vi "Autonomous Independent.vi"() -> ()   [LabVIEW 2013]
doc: "This VI is called when autonomous begins, and will automatically be terminated when autonomous ends. You can carry out timed or sensor driven robot movement independently without needing to return to the caller."
uses:
  <vilib>/Rock Robotics/WPI/DriverStation/WPI_DriverStationMatch Info.ctl
  <vilib>/Rock Robotics/WPI/Solenoid/WPI_SolenoidValue.ctl
  <vilib>/Rock Robotics/WPI/Relay/WPI_RelayValue.ctl
  Robot Global Data.vi
  <vilib>/addons/control/pid/pid.llb/PID (DBL).vi
  <vilib>/Rock Robotics/WPI/Solenoid/WPI_SolenoidSetEnum.vi
  <vilib>/Rock Robotics/WPI/Joystick/WPI_JoystickGetSetRefNum.vi
  <vilib>/addons/control/pid/NI_PID_pid.lvlib
panel:
  in  "Angle to Move Left":dbl=-1.1
  in  "Angle to Move Right":dbl=1.1 format="%.2f"
  in  "Feet To Move Left":dbl=2.0
  in  "Feet To Move Right":dbl=2.0 format="%.2f"
  out "Reseting constant":bool
  in  "Threshold for shooter":dbl=0.015
  out "Ready To Fire":bool
  in  "PID gains":T1={"proportional gain (Kc)"=1.0, "integral time (Ti, min)"=0.007, "derivative time (Td, min)"=0.0} {"derivative time (Td, min)" format="%.3f"; "integral time (Ti, min)" format="%.3f"; "proportional gain (Kc)" format="%.3f"}
  in  "Maximum Encoder speed":dbl=25000.0
  out "Time Last Fired":dbl
  in  "Posistioned":string="Nothing"
  in  "S Wait Time":dbl=1200.0
  in  "S Fire Time":dbl=1400.0
  in  "Shooter Speed":dbl format="%.2f"
  in  "Shooter On":bool=TRUE
  in  "Match Info":T2={"Autonomous Elapsed Seconds"=0.0, "TeleOp Elapsed Seconds"=0.0, "Disabled Elapsed Seconds"=0.0, "Visited Autonomous"=FALSE, "Visited TeleOp"=FALSE, "Visited Disabled"=FALSE, "Autonomous Settings"={"Autonomous Style"=enum."Independent", "VI Refnum"=refnum}}
  out "Angle Target":dbl
  out "Distance From Target":dbl
  in  "Current Status":string="Roaming"
  # "Be sure to right-click and choose Data Operations>>Make Current Value default if you want to save the array values with the VI"
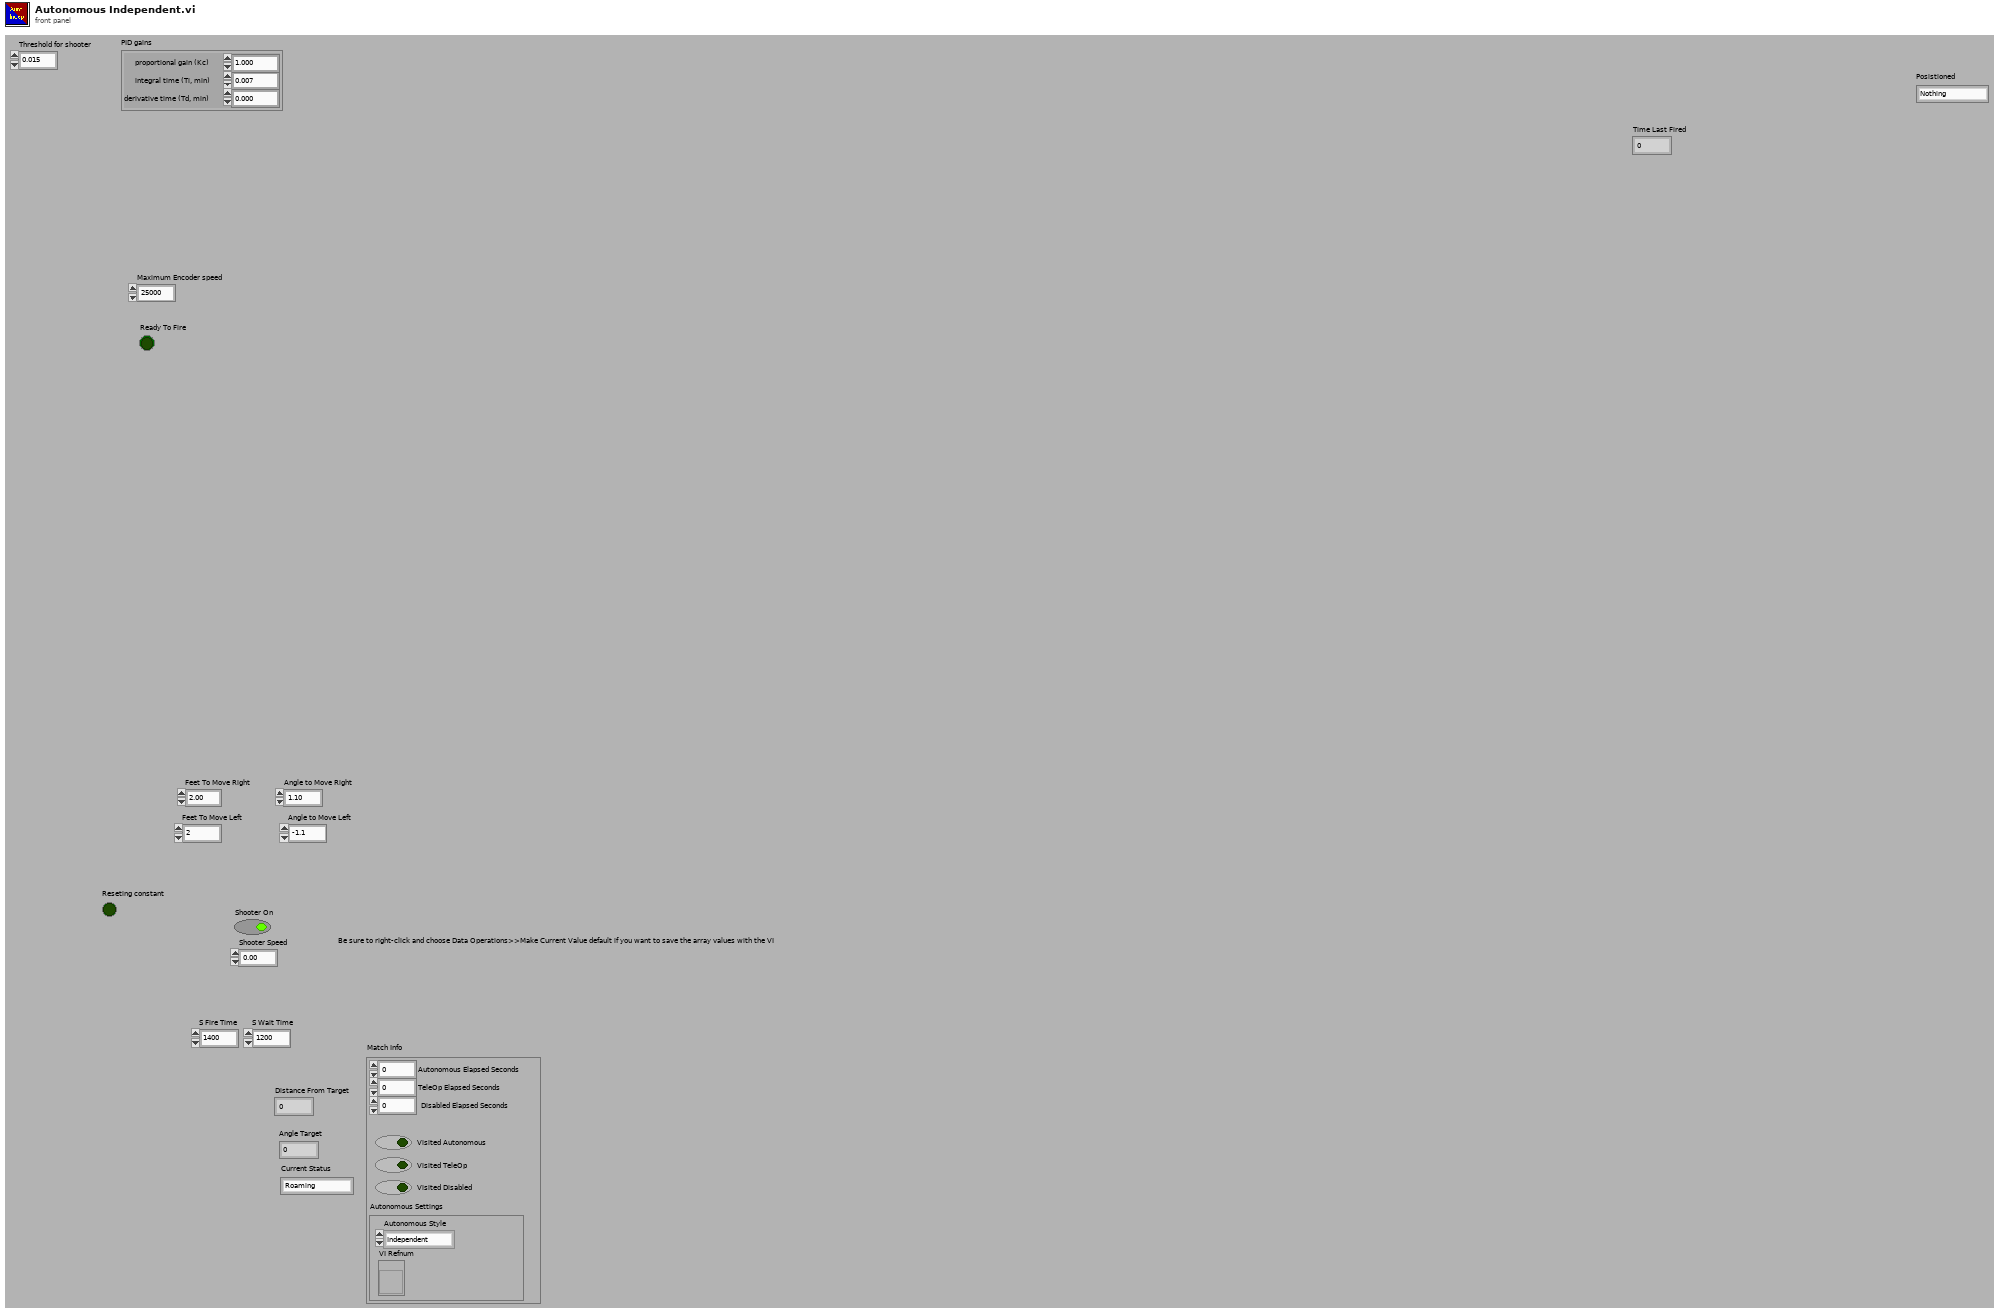
[diagram p1: front panel]
types:
  T1 = cluster{"proportional gain (Kc)":dbl, "integral time (Ti, min)":dbl, "derivative time (Td, min)":dbl}
  T2 = typedef "WPI_DriverStationMatch Info.ctl" = cluster{"Autonomous Elapsed Seconds":dbl, "TeleOp Elapsed Seconds":dbl, "Disabled Elapsed Seconds":dbl, "Visited Autonomous":bool, "Visited TeleOp":bool, "Visited Disabled":bool, "Autonomous Settings":cluster{"Autonomous Style":enum16{"Iterative", "Independent"}, "VI Refnum":refnum<vi>}}
  T3 = typedef "WPI_SolenoidValue.ctl" = enum16{"Off", "On", "Forward", "Reverse"}
  T4 = typedef "WPI_RelayValue.ctl" = enum16{"Off", "On", "Forward", "Reverse"}
  T5 = typedef "WPI_EncoderDevRef.ctl" = cluster{"DevStatus":errorcluster, "EncoderIndex":T6, "CounterIndex":T7, "DistancePerCount":dbl, "Decoding Type":T8}
  T6 = typedef "FPGA_EncoderIdx.ctl" = enum8{"Enc 0", "Enc 1", "Enc 2", "Enc 3", "Invalid"}
  T7 = typedef "FPGA_CounterCtrSystemIndex.ctl" = enum8{"Ctr 0", "Ctr 1", "Ctr 2", "Ctr 3", "Ctr 4", "Ctr 5", "Ctr 6", "Ctr 7", "Invalid"}
  T8 = typedef "WPI_EncoderType.ctl" = enum16{"1x", "2x", "4x"}
  T9 = typedef "WPI_RelayDevRef.ctl" = cluster{"DevStatus":errorcluster, "Relay Channel":T10, "Digital Module":T11, "Relay Direction":T12}
  T10 = typedef "FPGA_DIORelayChannel.ctl" = enum8{"Relay 1", "Relay 2", "Relay 3", "Relay 4", "Relay 5", "Relay 6", "Relay 7", "Relay 8", "Invalid"}
  T11 = typedef "FPGA_TypedefDigitalModule.ctl" = enum16{"Digital Module 1", "Digital Module 2"}
  T12 = typedef "WPI_RelayDirection.ctl" = enum16{"Both directions", "Forward only", "Reverse only"}
  T13 = typedef "WPI_SolenoidDevRef.ctl" = cluster{"DevStatus":errorcluster, "Solenoid Module":T14, "Forward Solenoid Channel":T15, "Reverse Solenoid Channel":T15}
  T14 = typedef "FPGA_TypedefSolenoidModule.ctl" = enum16{"Solenoid Module 1", "Solenoid Module 2"}
  T15 = typedef "WPI_SolenoidChannel.ctl" = enum8{"Solenoid 1", "Solenoid 2", "Solenoid 3", "Solenoid 4", "Solenoid 5", "Solenoid 6", "Solenoid 7", "Solenoid 8", "Invalid"}
  T16 = cluster{"Center Position":cluster{"X":dbl, "Y":dbl}, "Distance (ft)":dbl, "Center":bool}[]
  T17 = cluster{"Center Position":cluster{"X":dbl, "Y":dbl}, "Distance (ft)":dbl, "Center":bool}
  T18 = typedef "WPI_MotorControlDeviceRef.ctl" = cluster{"DeviceStatus":errorcluster, "Type":enum16{"PWM", "CAN"}, "PWM":cluster{"Digital Module":T11, "PWM Channel":T19, "DeadBand":T20}, "CAN":cluster{"Device Number":u8, "Control Mode":T21, "Semaphore":T22, "Max Vout":dbl}, "Invert":bool, "TransformRef":T23, "InvTransformRef":T23}
  T19 = typedef "FPGA_DIOPWMChannel.ctl" = enum8{"PWM 1", "PWM 2", "PWM 3", "PWM 4", "PWM 5", "PWM 6", "PWM 7", "PWM 8", "PWM 9", "PWM 10", "Invalid"}
  T20 = typedef "WPI_PWMDeadband.ctl" = cluster{"Name":string, "maxPositivePwm":i32, "minPositivePwm":i32, "centerPwm":i32, "maxNegativePwm":i32, "minNegativePwm":i32, "angularRange":u16}
  T21 = typedef "WPI_CANJaguar_ControlMode.ctl" = enum8{"Percent VBus", "Current", "Speed", "Position", "Voltage"}
  T22 = typedef "Semaphore RefNum" = refnum<k1>
  T23 = typedef "WPI_PWMTransform_ConPane.ctl" = refnum<vi>
  T24 = typedef "WPI_JoystickDevRef.ctl" = cluster{"Device":T25}
  T25 = typedef "WPI_JoystickDeviceEnum.ctl" = enum16{"USB 1", "USB 2", "USB 3", "USB 4", "Kinect 1", "Kinect 2"}
  T26 = cluster{"axis 1 (x)":dbl, "axis 2 (y)":dbl, "axis 3 (throttle)":dbl, "axis 4":dbl, "axis 5":dbl, "axis 6":dbl}
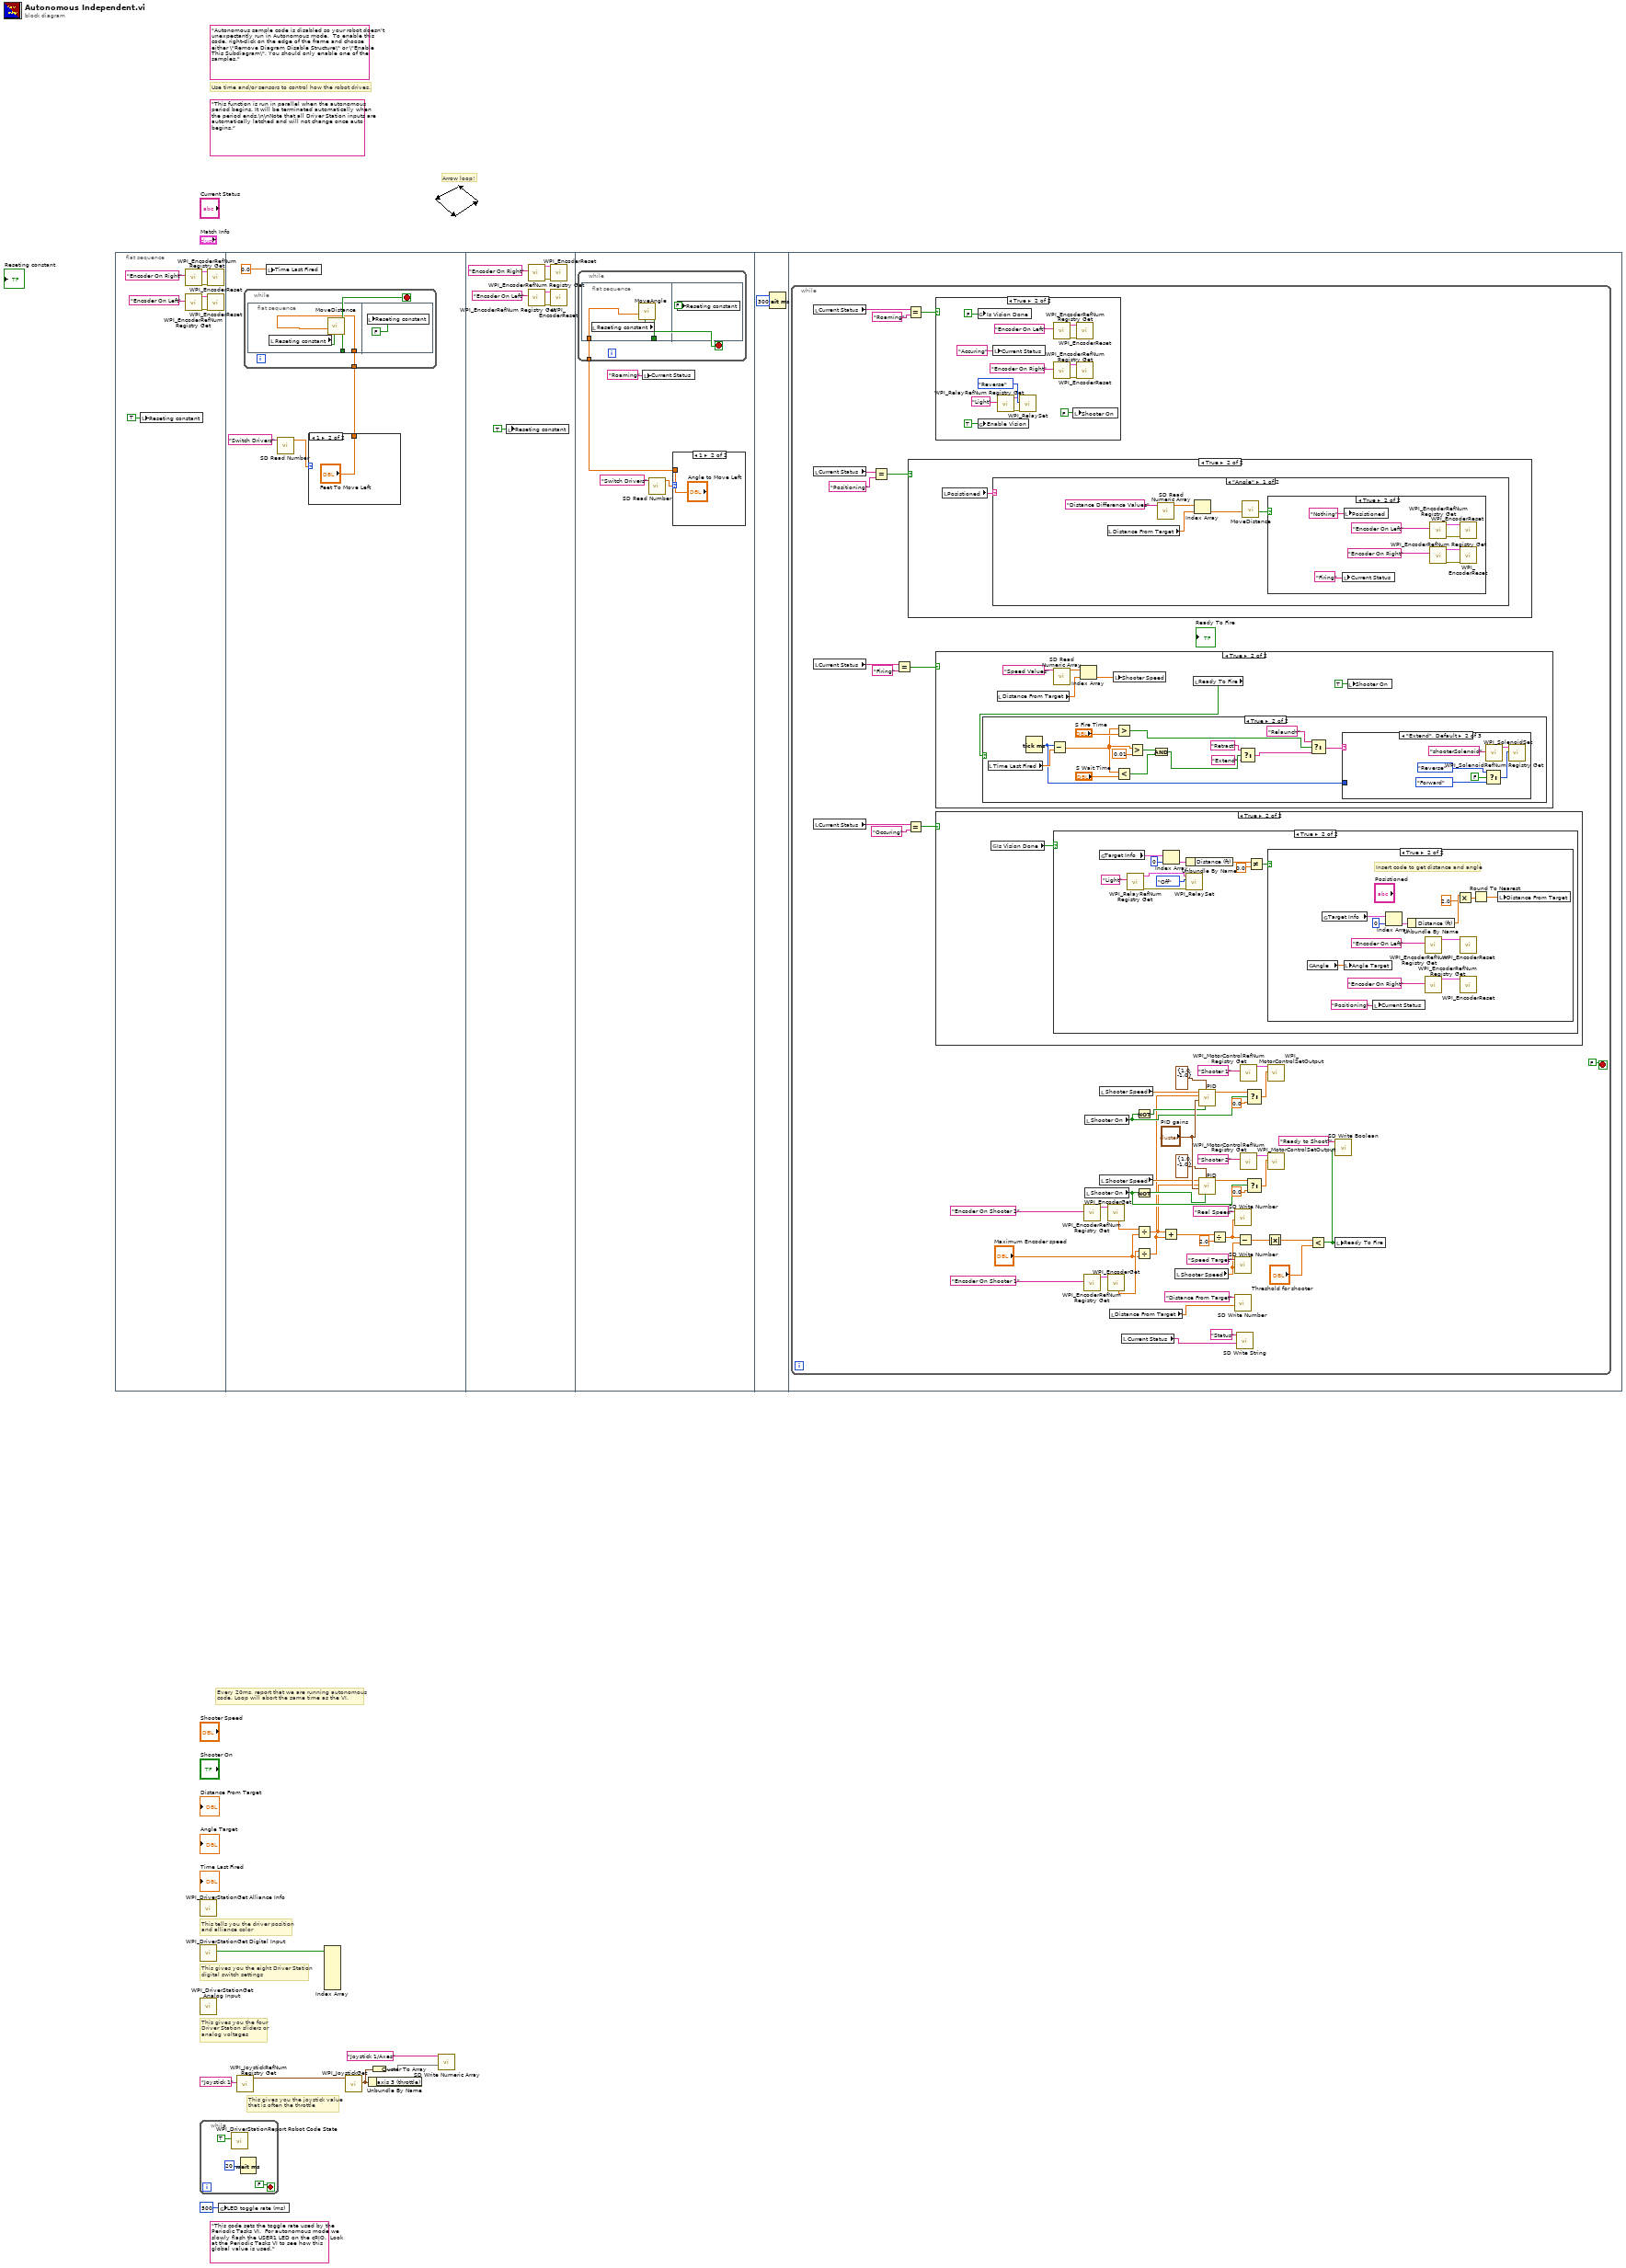
[diagram p0: block diagram]
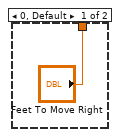
[diagram p2: hidden frame]
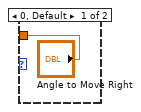
[diagram p3: hidden frame]
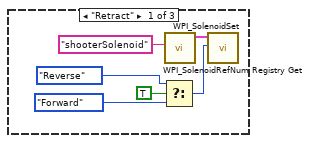
[diagram p6: hidden frame]
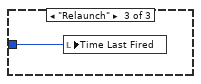
[diagram p7: hidden frame]
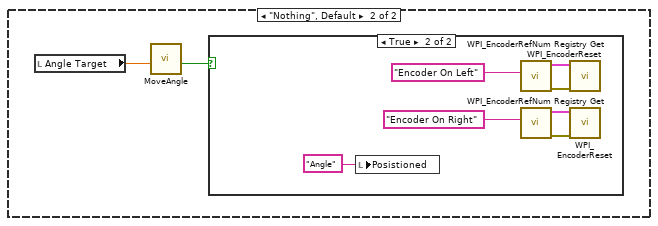
[diagram p11: hidden frame]
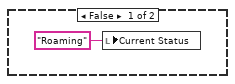
[diagram p15: hidden frame]
diagram:
  (unwired) "This code sets the toggle rate used by the Periodic Tasks VI.  For autonomous mode we slowly flash the USER1 LED on the cRIO.  Look at the Periodic Tasks VI to see how this global value is used."
  (unwired) "Autonomous sample code is disabled so your robot doesn't unexpectantly run in Autonomous mode.  To enable this code, right-click on the edge of the frame and choose either \"Remove Diagram Disable Structure\" or \"Enable This Subdiagram\". You should only enable one of the samples."
  (unwired) "This function is run in parallel when the autonomous period begins. It will be terminated automatically when the period ends.\n\nNote that all Driver Station inputs are automatically latched and will not change once auto begins."
  # "Arrow loop!"
  # "Every 20ms, report that we are running autonomous\ncode. Loop will abort the same time as the VI."
  # "This gives you the joystick value\nthat is often the throttle"
  # "Use time and/or sensors to control how the robot drives."
  # "This tells you the driver position\nand alliance color"
  # "This gives you the eight Driver Station\ndigital switch settings"
  # "This gives you the four\nDriver Station sliders or\nanalog voltages"
  n1 = flat-sequence {
    frame #0 {
      n2 = local write "Reseting constant"(TRUE ("Reseting constant")) -> ()
      n3 = call <vilib>:"WPI_EncoderRefNum Registry Get.vi"("refnum name"="Encoder On Right") -> ("error out"=w9:errorcluster, "EncoderDevRef"=w10:T5)  [unwired: 9 in]
      n4 = call <vilib>:"WPI_EncoderRefNum Registry Get.vi"("refnum name"="Encoder On Left") -> ("error out"=w11:errorcluster, "EncoderDevRef"=w12:T5)  [unwired: 9 in]
      n5 = call <vilib>:"WPI_EncoderReset.vi"("error in (no error)"=w9, "EncoderDevRef"=w10) -> ()  [unwired: 8 in, 2 out]
      n6 = call <vilib>:"WPI_EncoderReset.vi"("error in (no error)"=w11, "EncoderDevRef"=w12) -> ()  [unwired: 8 in, 2 out]
    }
    frame #1 {
      n7 = local write "Time Last Fired"(0.0 ("Time Last Fired")) -> ()
      n8 = call <vilib>:"SD Read Number.vi"("Name"="Switch Drivers") -> ("Numeric"=w16:dbl)  [unwired: 8 in, 2 out]
      n9 = case shown="1" w16 {
        tunnel: ["Feet To Move Right" "Feet To Move Left"] -> w15
        frame 0, Default {
        }
        frame 1 {
        }
      }
      n10 = while {
        tunnel: w15 -> [w21]
        stop <- w22 stop-if-true
        n11 = flat-sequence {
          tunnel: [w25] -> w22
          tunnel: w21 -> [w23]
          frame #0 {
            n12 = local read "Reseting constant"() -> (w24:bool)
            n13 = call "MoveDistance.vi"("reinitialize? (F)"=w24, "Distance From Target"=w23) -> ("Done?"=w25:bool)  [unwired: 9 in]
          }
          frame #1 {
            n14 = local write "Reseting constant"(FALSE ("Reseting constant")) -> ()
          }
        }
      }
    }
    frame #2 {
      n15 = local write "Reseting constant"(TRUE ("Reseting constant")) -> ()
      n16 = call <vilib>:"WPI_EncoderRefNum Registry Get.vi"("refnum name"="Encoder On Right") -> ("error out"=w33:errorcluster, "EncoderDevRef"=w32:T5)  [unwired: 9 in]
      n17 = call <vilib>:"WPI_EncoderRefNum Registry Get.vi"("refnum name"="Encoder On Left") -> ("error out"=w31:errorcluster, "EncoderDevRef"=w30:T5)  [unwired: 9 in]
      n18 = call <vilib>:"WPI_EncoderReset.vi"("error in (no error)"=w33, "EncoderDevRef"=w32) -> ()  [unwired: 8 in, 2 out]
      n19 = call <vilib>:"WPI_EncoderReset.vi"("error in (no error)"=w31, "EncoderDevRef"=w30) -> ()  [unwired: 8 in, 2 out]
    }
    frame #3 {
      n20 = local write "Current Status"("Roaming" ("Current Status")) -> ()
      n21 = call <vilib>:"SD Read Number.vi"("Name"="Switch Drivers") -> ("Numeric"=w35:dbl)  [unwired: 8 in, 2 out]
      n22 = case shown="1" w35 {
        tunnel: ["Angle to Move Right" "Angle to Move Left"] -> w34
        frame 0, Default {
        }
        frame 1 {
        }
      }
      n23 = while {
        tunnel: w34 -> [w40]
        stop <- w41 stop-if-true
        n24 = flat-sequence {
          tunnel: [w44] -> w41
          tunnel: w40 -> [w42]
          frame #0 {
            n25 = local read "Reseting constant"() -> (w43:bool)
            n26 = call "MoveAngle.vi"("reinitialize? (F)"=w43, "Angle Target"=w42) -> ("Done?"=w44:bool)  [unwired: 9 in]
          }
          frame #1 {
            n27 = local write "Reseting constant"(FALSE ("Reseting constant")) -> ()
          }
        }
      }
    }
    frame #4 {
      n28 = Wait (ms)(milliseconds to wait=u32 300) -> ()  [unwired: 1 out]
    }
    frame #5 {
      n29 = while {
        stop <- FALSE stop-if-true
        n30 = local read "Current Status"() -> (w94:string)
        n31 = local read "Current Status"() -> (w98:string)
        n32 = local read "Current Status"() -> (w91:string)
        n33 = local read "Current Status"() -> (w102:string)
        n34 = Equal?(x=w98, y="Positioning") -> (x = y?=w96:bool)
        n35 = Equal?(x=w91, y="Firing") -> (x = y?=w92:bool)
        n36 = Equal?(x=w94, y="Roaming") -> (x = y?=w93:bool)
        n37 = Equal?(x=w102, y="Occuring") -> (x = y?=w100:bool)
        n38 = case shown="True" w96 {
          frame False {
          }
          frame True {
            n39 = local read "Posistioned"() -> (w151:string)
            n40 = case shown="\"Angle\"" w151 {
              frame "Angle" {
                n41 = local read "Distance From Target"() -> (w154:dbl)
                n42 = call <vilib>:"SD Read Numeric Array.vi"("Name"="Distance Difference Values") -> ("Numeric Array"=w156:dbl[])  [unwired: 8 in, 2 out]
                n43 = Index Array(array=w156, index=w154) -> (element=w153:dbl)
                n44 = call "MoveDistance.vi"("Distance From Target"=w153) -> ("Done?"=w152:bool)  [unwired: 10 in]
                n45 = case shown="True" w152 {
                  frame False {
                  }
                  frame True {
                    n46 = local write "Current Status"("Firing" ("Current Status")) -> ()
                    n47 = local write "Posistioned"("Nothing" ("Posistioned")) -> ()
                    n48 = call <vilib>:"WPI_EncoderRefNum Registry Get.vi"("refnum name"="Encoder On Left") -> ("error out"=w160:errorcluster, "EncoderDevRef"=w161:T5)  [unwired: 9 in]
                    n49 = call <vilib>:"WPI_EncoderRefNum Registry Get.vi"("refnum name"="Encoder On Right") -> ("error out"=w162:errorcluster, "EncoderDevRef"=w163:T5)  [unwired: 9 in]
                    n50 = call <vilib>:"WPI_EncoderReset.vi"("error in (no error)"=w160, "EncoderDevRef"=w161) -> ()  [unwired: 8 in, 2 out]
                    n51 = call <vilib>:"WPI_EncoderReset.vi"("error in (no error)"=w162, "EncoderDevRef"=w163) -> ()  [unwired: 8 in, 2 out]
                  }
                }
              }
              frame "Nothing", Default {
                n52 = local read "Angle Target"() -> (w166:dbl)
                n53 = call "MoveAngle.vi"("Angle Target"=w166) -> ("Done?"=w165:bool)  [unwired: 10 in]
                n54 = case shown="True" w165 {
                  frame False {
                  }
                  frame True {
                    n55 = local write "Posistioned"("Angle" ("Posistioned")) -> ()
                    n56 = call <vilib>:"WPI_EncoderRefNum Registry Get.vi"("refnum name"="Encoder On Left") -> ("error out"=w171:errorcluster, "EncoderDevRef"=w170:T5)  [unwired: 9 in]
                    n57 = call <vilib>:"WPI_EncoderRefNum Registry Get.vi"("refnum name"="Encoder On Right") -> ("error out"=w169:errorcluster, "EncoderDevRef"=w168:T5)  [unwired: 9 in]
                    n58 = call <vilib>:"WPI_EncoderReset.vi"("error in (no error)"=w171, "EncoderDevRef"=w170) -> ()  [unwired: 8 in, 2 out]
                    n59 = call <vilib>:"WPI_EncoderReset.vi"("error in (no error)"=w169, "EncoderDevRef"=w168) -> ()  [unwired: 8 in, 2 out]
                  }
                }
              }
            }
          }
        }
        n60 = case shown="True" w93 {
          frame False {
          }
          frame True {
            n61 = global write "Robot Global Data.vi" "Is Vision Done"(FALSE ("Is Vision Done")) -> ()
            n62 = global write "Robot Global Data.vi" "Enable Vision"(TRUE ("Enable Vision")) -> ()
            n63 = local write "Current Status"("Accuring" ("Current Status")) -> ()
            n64 = call <vilib>:"WPI_RelayRefNum Registry Get.vi"("refnum name"="Light") -> ("error out"=w148:errorcluster, "RelayDevRef"=w147:T9)  [unwired: 9 in]
            n65 = call <vilib>:"WPI_RelaySet.vi"("error in (no error)"=w148, "RelayValue"=WPI_RelayValue."Reverse", "RelayDevRef"=w147) -> ()  [unwired: 7 in, 2 out]
            n66 = call <vilib>:"WPI_EncoderRefNum Registry Get.vi"("refnum name"="Encoder On Left") -> ("error out"=w142:errorcluster, "EncoderDevRef"=w141:T5)  [unwired: 9 in]
            n67 = call <vilib>:"WPI_EncoderRefNum Registry Get.vi"("refnum name"="Encoder On Right") -> ("error out"=w144:errorcluster, "EncoderDevRef"=w143:T5)  [unwired: 9 in]
            n68 = local write "Shooter On"(FALSE ("Shooter On")) -> ()
            n69 = call <vilib>:"WPI_EncoderReset.vi"("error in (no error)"=w142, "EncoderDevRef"=w141) -> ()  [unwired: 8 in, 2 out]
            n70 = call <vilib>:"WPI_EncoderReset.vi"("error in (no error)"=w144, "EncoderDevRef"=w143) -> ()  [unwired: 8 in, 2 out]
          }
        }
        n71 = case shown="True" w92 {
          frame False {
          }
          frame True {
            n72 = local read "Distance From Target"() -> (w105:dbl)
            n73 = call <vilib>:"SD Read Numeric Array.vi"("Name"="Speed Values") -> ("Numeric Array"=w107:dbl[])  [unwired: 8 in, 2 out]
            n74 = Index Array(array=w107, index=w105) -> (element=w106:dbl)
            n75 = local write "Shooter Speed"(w106) -> ()
            n76 = local read "Ready To Fire"() -> (w104:bool)
            n77 = case shown="True" w104 {
              frame False {
              }
              frame True {
                n78 = local read "Time Last Fired"() -> (w123:dbl)
                n79 = Tick Count (ms)() -> (millisecond timer value=w111:u32)
                n80 = Subtract(x=w111, y=w123) -> (x-y=w116:dbl)
                n81 = Greater?(x=w116, y="S Fire Time") -> (0:w119:bool)
                n82 = Less?(x=w116, y="S Wait Time") -> (x < y?=w113:bool)
                n83 = Greater?(x=w116, y=0.01) -> (0:w114:bool)
                n84 = And(x=w114, y=w113) -> (x .and. y?=w112:bool)
                n85 = Select(t="Retract" ("f"), s=w112, f="Extend") -> (s? t:f=w117:string)
                n86 = Select(t="Relaunch" ("f"), s=w119, f=w117) -> (s? t:f=w121:string)
                n87 = case shown="\"Extend\", Default" w121 {
                  tunnel: w111 -> [_ _ w136]
                  frame "Retract" {
                    n88 = Select(t=WPI_SolenoidValue."Reverse" ("Value"), s=TRUE, f=WPI_SolenoidValue."Forward" ("Value")) -> (s? t:f=w128:T3)
                    n89 = call <vilib>:"WPI_SolenoidRefNum Registry Get.vi"("refnum name"="shooterSolenoid") -> ("SolenoidDevRef"=w124:T13)  [unwired: 9 in, 1 out]
                    n90 = call-poly <vilib>:"WPI_SolenoidSet.vi"("Value"=w128, "SolenoidDevRef"=w124) -> ()  [unwired: 8 in, 2 out]
                  }
                  frame "Extend", Default {
                    n91 = Select(t=WPI_SolenoidValue."Reverse" ("Value"), s=FALSE, f=WPI_SolenoidValue."Forward" ("Value")) -> (s? t:f=w134:T3)
                    n92 = call <vilib>:"WPI_SolenoidRefNum Registry Get.vi"("refnum name"="shooterSolenoid") -> ("SolenoidDevRef"=w130:T13)  [unwired: 9 in, 1 out]
                    n93 = call-poly <vilib>:"WPI_SolenoidSet.vi"("Value"=w134, "SolenoidDevRef"=w130) -> ()  [unwired: 8 in, 2 out]
                  }
                  frame "Relaunch" {
                    n94 = local write "Time Last Fired"(w136) -> ()
                  }
                }
              }
            }
            n95 = local write "Shooter On"(TRUE ("Shooter On")) -> ()
          }
        }
        n96 = case shown="True" w100 {
          frame False {
          }
          frame True {
            n97 = global read "Robot Global Data.vi" "Is Vision Done"() -> (w174:bool)
            n98 = case shown="True" w174 {
              frame False {
              }
              frame True {
                n99 = global read "Robot Global Data.vi" "Target Info"() -> (w184:T16)
                n100 = call <vilib>:"WPI_RelayRefNum Registry Get.vi"("refnum name"="Light") -> ("error out"=w177:errorcluster, "RelayDevRef"=w178:T9)  [unwired: 9 in]
                n101 = Index Array(array=w184, index=0) -> (element=w182:T17)
                n102 = Unbundle By Name(w182) -> ("Distance (ft)"=w180:dbl)
                n103 = call <vilib>:"WPI_RelaySet.vi"("error in (no error)"=w177, "RelayValue"=WPI_RelayValue."Off", "RelayDevRef"=w178) -> ()  [unwired: 7 in, 2 out]
                n104 = Not Equal?(x=w180, y=0.0) -> (x != y?=w181:bool)
                n105 = case shown="True" w181 {
                  frame False {
                    n106 = local write "Current Status"("Roaming" ("Current Status")) -> ()
                  }
                  frame True {
                    # "Insert code to get distance and angle"
                    n107 = global read "Robot Global Data.vi" "Angle"() -> (w193:dbl)
                    n108 = global read "Robot Global Data.vi" "Target Info"() -> (w192:T16)
                    n109 = local write "Angle Target"(w193) -> ()
                    n110 = local write "Current Status"("Positioning" ("Current Status")) -> ()
                    n111 = Index Array(array=w192, index=0) -> (element=w190:T17)
                    n112 = Unbundle By Name(w190) -> ("Distance (ft)"=w188:dbl)
                    n113 = call <vilib>:"WPI_EncoderRefNum Registry Get.vi"("refnum name"="Encoder On Left") -> ("EncoderDevRef"=w196:T5)  [unwired: 9 in, 1 out]
                    n114 = call <vilib>:"WPI_EncoderRefNum Registry Get.vi"("refnum name"="Encoder On Right") -> ("EncoderDevRef"=w195:T5)  [unwired: 9 in, 1 out]
                    n115 = Multiply(x=w188, y=2.0) -> (x*y=w186:dbl)
                    n116 = call <vilib>:"WPI_EncoderReset.vi"("EncoderDevRef"=w196) -> ()  [unwired: 9 in, 2 out]
                    n117 = call <vilib>:"WPI_EncoderReset.vi"("EncoderDevRef"=w195) -> ()  [unwired: 9 in, 2 out]
                    n118 = Round To Nearest(number=w186) -> (nearest integer value=w189:dbl)
                    n119 = local write "Distance From Target"(w189) -> ()
                  }
                }
              }
            }
          }
        }
        n120 = call <vilib>:"WPI_EncoderRefNum Registry Get.vi"("refnum name"="Encoder On Shooter 2") -> ("EncoderDevRef"=w77:T5)  [unwired: 9 in, 1 out]
        n121 = call <vilib>:"WPI_EncoderRefNum Registry Get.vi"("refnum name"="Encoder On Shooter 1") -> ("EncoderDevRef"=w86:T5)  [unwired: 9 in, 1 out]
        n122 = local read "Shooter On"() -> (w66:bool)
        n123 = local read "Shooter On"() -> (w67:bool)
        n124 = local read "Shooter Speed"() -> (w65:dbl)
        n125 = local read "Shooter Speed"() -> (w64:dbl)
        n126 = call <vilib>:"WPI_EncoderGet.vi"("EncoderDevRef"=w77) -> ("Rate"=w69:dbl)  [unwired: 5 in, 5 out]
        n127 = call <vilib>:"WPI_EncoderGet.vi"("EncoderDevRef"=w86) -> ("Rate"=w70:dbl)  [unwired: 5 in, 5 out]
        n128 = local read "Distance From Target"() -> (w48:dbl)
        n129 = local read "Current Status"() -> (w47:string)
        n130 = Not(x=w66) -> (.not. x?=w88:bool)
        n131 = Not(x=w67) -> (.not. x?=w79:bool)
        n132 = Divide(x=w69, y="Maximum Encoder speed") -> (x/y=w62:dbl)
        n133 = Divide(x=w70, y="Maximum Encoder speed") -> (x/y=w61:dbl)
        n134 = Add(x=w62, y=w61) -> (x+y=w60:dbl)
        n135 = local read "Shooter Speed"() -> (w57:dbl)
        n136 = call-poly <vilib>:"PID.vi"("reinitialize? (F)"=w88, "output range"=cluster{"output high":dbl, "output low":dbl} {"output high"=1.0, "output low"=-1.0}, "PID gains"="PID gains", "process variable"=w61, "setpoint"=w65) -> ("output"=w87:dbl)  [unwired: 5 in, 1 out]
        n137 = call-poly <vilib>:"PID.vi"("reinitialize? (F)"=w79, "output range"=cluster{"output high":dbl, "output low":dbl} {"output high"=1.0, "output low"=-1.0}, "PID gains"="PID gains", "process variable"=w62, "setpoint"=w64) -> ("output"=w78:dbl)  [unwired: 5 in, 1 out]
        n138 = Divide(x=w60, y=2.0) -> (x/y=w56:dbl)
        n139 = call <vilib>:"SD Write Number.vi"("Numeric"=w48, "Name"="Distance From Target") -> ()  [unwired: 8 in, 2 out]
        n140 = call <vilib>:"SD Write Number.vi"("Numeric"=w56, "Name"="Real Speed") -> ()  [unwired: 8 in, 2 out]
        n141 = call <vilib>:"SD Write Number.vi"("Numeric"=w57, "Name"="Speed Target") -> ()  [unwired: 8 in, 2 out]
        n142 = call <vilib>:"SD Write String.vi"("String"=w47, "Name"="Status") -> ()  [unwired: 8 in, 2 out]
        n143 = Subtract(x=w56, y=w57) -> (x-y=w55:dbl)
        n144 = call <vilib>:"WPI_MotorControlRefNum Registry Get.vi"("refnum name"="Shooter 1") -> ("MotorControlDevRef"=w81:T18)  [unwired: 9 in, 1 out]
        n145 = call <vilib>:"WPI_MotorControlRefNum Registry Get.vi"("refnum name"="Shooter 2") -> ("MotorControlDevRef"=w72:T18)  [unwired: 9 in, 1 out]
        n146 = Select(t=w87, s=w66, f=0.0) -> (s? t:f=w83:dbl)
        n147 = Select(t=w78, s=w67, f=0.0) -> (s? t:f=w74:dbl)
        n148 = Absolute Value(x=w55) -> (abs(x)=w54:dbl)
        n149 = call <vilib>:"WPI_MotorControlSetOutput.vi"("Output"=w83, "MotorControlDevRef"=w81) -> ()  [unwired: 7 in, 3 out]
        n150 = call <vilib>:"WPI_MotorControlSetOutput.vi"("Output"=w74, "MotorControlDevRef"=w72) -> ()  [unwired: 7 in, 3 out]
        n151 = Less?(x=w54, y="Threshold for shooter") -> (x < y?=w52:bool)
        n152 = call <vilib>:"SD Write Boolean.vi"("Boolean"=w52, "Name"="Ready to Shoot?") -> ()  [unwired: 8 in, 2 out]
        n153 = local write "Ready To Fire"(w52) -> ()
      }
    }
  }
  n154 = call <vilib>:"WPI_DriverStationGet Alliance Info.vi"() -> ()  [unwired: 12 out]
  n155 = call <vilib>:"WPI_DriverStationGet Digital Input.vi"() -> ("Driver Station Digital Input (1-8)"=w7:bool[])  [unwired: 11 out]
  n156 = call <vilib>:"WPI_DriverStationGet Analog Input.vi"() -> ()  [unwired: 12 out]
  n157 = while {
    stop <- FALSE stop-if-true
    n158 = call <vilib>:"WPI_DriverStationReport Robot Code State.vi"("Autonomous"=TRUE) -> ()  [unwired: 10 in, 1 out]
    n159 = Wait (ms)(milliseconds to wait=u32 20) -> ()  [unwired: 1 out]
  }
  n160 = global write "Robot Global Data.vi" "LED toggle rate (ms)"(u32 500 ("LED ms toggle rate")) -> ()
  n161 = call <vilib>:"WPI_JoystickRefNum Registry Get.vi"("refnum name"="Joystick 1") -> ("JoystickDevRef"=w5:T24)  [unwired: 1 in, 9 out]
  n162 = Index Array(array=w7) -> ()  [unwired: 8 in, 8 out]
  n163 = call <vilib>:"WPI_JoystickGet.vi"("JoystickDevRef"=w5) -> ("Axes"=w2:T26)  [unwired: 1 in, 5 out]
  n164 = Unbundle By Name(w2) -> ()  [unwired: 1 out]
  n165 = Cluster To Array(cluster=w2) -> (array=w3:dbl[])
  n166 = call <vilib>:"SD Write Numeric Array.vi"("Numeric Array"=w3, "Name"="Joystick 1/Axes") -> ()  [unwired: 8 in, 2 out]
